vi "Update Armed.vi"(8 "error in (no error)":errorcluster, 9 "Devices armed":bool[](array[boolean]), 10 "Armed":bool, 11 "Monitor-Pulse in":refnum<class "LabActor.lvclass">) -> (0 "error out":errorcluster, 3 "Monitor-Pulse out":refnum<class "LabActor.lvclass">)   [LabVIEW 2018, in "LabActor.lvclass"]
uses:
  LabActor.lvclass
  C:/github/LabActor/Controllers/Application Controller/Application Controller.lvclass
  Controllers/Application Controller/Application Controller.lvclass/Application Controller.ctl
  Controllers/Application Controller/Read Armed ref.vi
  Controllers/Application Controller/Read Devices armed.vi
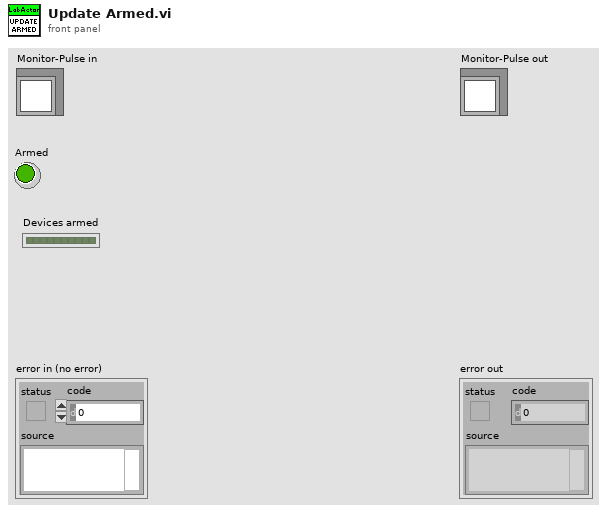
[diagram p1: front panel]
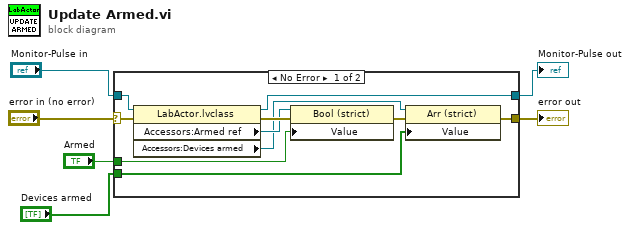
[diagram p0: block diagram]
diagram:
  n1 = case shown="No Error" "error in (no error)" {
    selector: "error in (no error)" -> [w15 w18]
    tunnel: [w8 w18] -> w5
    tunnel: [w12 w17] -> w3
    tunnel: "Monitor-Pulse in" -> [w13 w17]
    tunnel: "Armed" -> [w16 _]
    tunnel: "Devices armed" -> [w7 _]
    frame No Error {
      n2 = property class="LabActor.lvclass"(reference=w13, error in=w15) -> (reference out=w12:refnum<class "LabActor.lvclass">, error out=w14:errorcluster, "Accessors:Armed ref"=w11:refnum<vi>, "Accessors:Devices armed"=w10:refnum<vi>)
      n3 = property class="Bool (strict)"(reference=w11, error in=w14, "Value"=w16) -> (error out=w9:errorcluster)  [unwired: 1 out]
      n4 = property class="Arr (strict)"(reference=w10, error in=w9, "Value"=w7) -> (error out=w8:errorcluster)  [unwired: 1 out]
    }
    frame Error {
    }
  }
  "error out" <- w5
  "Monitor-Pulse out" <- w3
